vi "Rd Wr Filter Wheel Settings.vi"(7 "Wheel Name":string="Default", 8 "error in (no error)":errorcluster, 9 "Settings File":string="CC System Settings.json", 10 "Write? (F:Read)":bool, 11 "Filter Wheel Settings":T1={"Num Wheels"=0, "Filters"=[], "Invalid Combinations"=[], "Addr"="", "Name"="", "Simulate"=FALSE, "Homing Parameters"={"Direction (F: CW)"=TRUE, "Speed"=150, "Accel"=400, "Min Distance"=2700, "Short Leg"=0, "Error Cnts"=0}, "Default Speed"=200} {"Default Speed" min=20 max=4000 step=10}) -> (0 "error out":errorcluster, 3 "Filter Wheel Settings":T1={"Num Wheels"=0, "Filters"=[], "Invalid Combinations"=[], "Addr"="", "Name"="", "Simulate"=FALSE, "Homing Parameters"={"Direction (F: CW)"=TRUE, "Speed"=150, "Accel"=400, "Min Distance"=2700, "Short Leg"=0, "Error Cnts"=0}, "Default Speed"=1000} {"Default Speed" min=20 max=4000 step=10})   [LabVIEW 2021, in "Filter Wheel.lvclass"]
uses:
  Filter Wheel Object/Filter Wheel.lvclass
  Filter Wheel configuration.ctl
  Filter Wheel Object/Filter Wheel Details.ctl
  Filter Wheel Arduino Control/Filter Wheel Arduino Homing cluster.ctl
  65bd8ba7-6c5f-49c3-986f-02d69eb152e8.vi
  1ff77ff5-bc7f-48d0-940d-8d167d473090.vi
  <vilib>/JDP Science/JSONtext/Find Item.vi
  <vilib>/JDP Science/JSONtext/Next JSON Value.vi
  <vilib>/JDP Science/JSONtext/String Subset.vi
  <vilib>/JDP Science/JSONtext/Parsing/Advance past next JSON Value (inlined COPY).vi
  <vilib>/JDP Science/JSONtext/Parsing/Advance past whitespace.vi
  <vilib>/JDP Science/JSONtext/Parsing/Advance past String.vi
  <vilib>/JDP Science/JSONtext/Parsing/Advance past Number.vi
  <vilib>/JDP Science/JSONtext/Parsing/Advance past Line Ending.vi
  <vilib>/JDP Science/JSONtext/Parsing/Parse Full Path or Item Name.vi
  <vilib>/JDP Science/JSONtext/Parsing/Advance past Array.vi
  <vilib>/JDP Science/JSONtext/Parsing/Advance past Object.vi
  <vilib>/JDP Science/JSONtext/support/Error Cluster From Code.vi
  <vilib>/JDP Science/JSONtext/Offset/Find Item Locations by Path.vi
  <vilib>/JDP Science/JSONtext/JSON text to Variant.vi
  <vilib>/JDP Science/JSONtext/Variant to JSON Text.vi
  <vilib>/JDP Science/JSONtext/Set Item.vi
  <vilib>/JDP Science/JSONtext/LVClass Serializer/JSONtext LVClass Serializer.lvclass
  <vilib>/JDP Science/JSONtext/JSONtext.lvlib
panel:
  out "<JSON>":string caption="JSON"
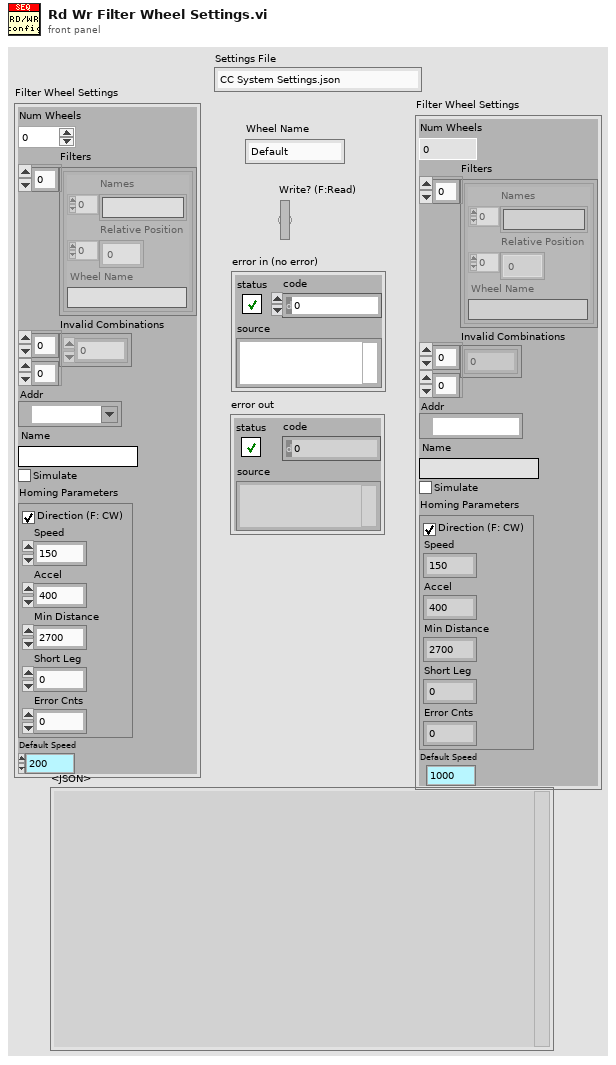
[diagram p1: front panel]
types:
  T1 = typedef "Filter Wheel.lvclass/Filter Wheel configuration.ctl" = cluster{"Num Wheels":i32, "Filters":T2[], "Invalid Combinations":i32[][], "Addr":refnum<visa-resource-name>, "Name":string, "Simulate":bool, "Homing Parameters":T3, "Default Speed":u16}
  T2 = typedef "Filter Wheel.lvclass/Filter Wheel Details.ctl" = cluster{"Names":string[], "Relative Position":i32[], "Wheel Name":string}
  T3 = typedef "Filter Wheel Arduino Homing cluster.ctl" = cluster{"Direction (F: CW)":bool, "Speed":i32, "Accel":i32, "Min Distance":i32, "Short Leg":i32, "Error Cnts":i32}
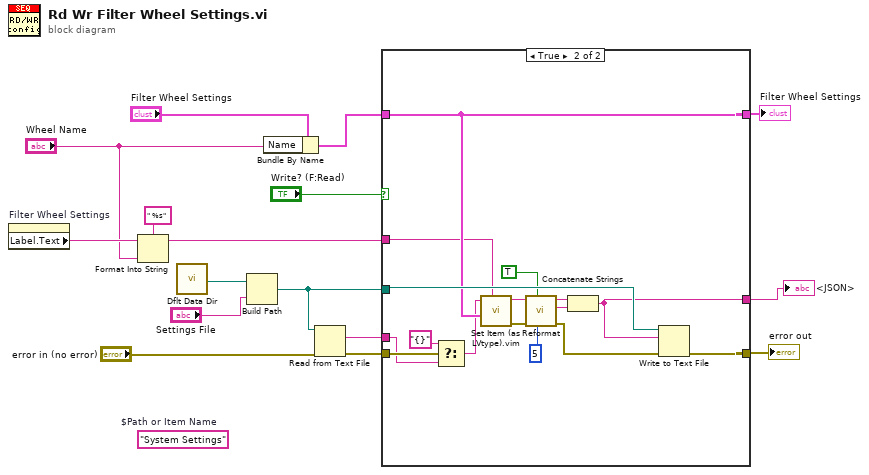
[diagram p0: block diagram]
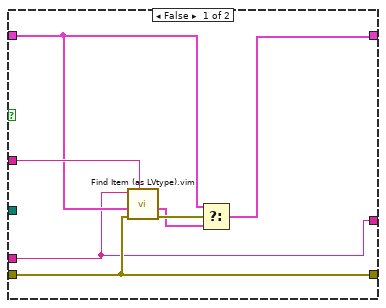
[diagram p2: hidden frame]
diagram:
  (unwired) "System Settings"  # $Path or Item Name
  n1 = property on="Filter Wheel Settings" class="Clust (strict)"() -> ("Label.Text"=w5:string)  [unwired: 2 in, 2 out]
  n2 = Format Into String(format string=" %s", initial string=w5, "Wheel Name") -> (resulting string=w2:string)  [unwired: 1 in, 1 out]
  n3 = call <vilib>:"Dflt Data Dir.vi"() -> ("App:Default Data Directory"=w16:path)
  n4 = Build Path(base path=w16, name or relative path="Settings File") -> (appended path=w12:path)
  n5 = Bundle By Name(cluster="Filter Wheel Settings", "Name"="Wheel Name") -> (w3:T1)
  n6 = Read from Text File(file (use dialog)=w12, error in="error in (no error)") -> (text=w13:string, error out=w14:errorcluster)  [unwired: 2 in, 2 out]
  n7 = case shown="True" "Write? (F:Read)" {
    tunnel: w14 -> [w18 w35]
    tunnel: w3 -> [w21 w37]
    tunnel: w12 -> [_ w39]
    tunnel: [w18 w38] -> w10
    tunnel: [w23 w37] -> w11
    tunnel: w2 -> [w22 w36]
    tunnel: w13 -> [w17 w33]
    tunnel: [w17 w25] -> w7
    frame False {
      n8 = call "Find Item (as LVtype).vim"("$Path or Item Name"=w22, "error in (no error)"=w18, "Data Type and Default Value"=w21, "JSON"=w17) -> ("error out"=w20:errorcluster, "Data"=w19:T1)  [unwired: 4 in, 2 out]
      n9 = Select(t=w21, s=w20, f=w19) -> (s? t:f=w23:T1)
    }
    frame True {
      n10 = Select(t="{}" ("JSON"), s=w35, f=w33) -> (s? t:f=w32:string)
      n11 = call "Set Item (as LVtype).vim"("$Path or Item Name"=w36, "Anything"=w37, "JSON"=w32) -> ("error out"=w29:errorcluster, "<JSON>"=w30:string)  [unwired: 5 in, 1 out]
      n12 = call <vilib>:"Reformat.vi"("Pretty Print Levels"=5, "Alphabetically Sort Objects"=TRUE, "error in (no error)"=w29, "JSON"=w30) -> ("error out"=w28:errorcluster, "Rest of Input String"=w24:string, "<JSON>"=w27:string)  [unwired: 4 in, 1 out]
      n13 = Concatenate Strings(w27, w24) -> (w25:string)
      n14 = Write to Text File(file (use dialog)=w39, text=w25, error in=w28) -> (error out=w38:errorcluster)  [unwired: 1 in, 2 out]
    }
  }
  "error out" <- w10
  "Filter Wheel Settings" <- w11
  "<JSON>" <- w7
